vi "measure_mpps.vi"(0 "User Name":string, 1 "Cell details cluster":T2={"Cell Position"=16, "Cell Label"="", "Pixel to measure"=0, "Area (cm^2)"=0.126, "Variable"="", "Variable value"="", "Scan settings in queue"=0, "Light or dark"="", "Measurement Type"=""} {"Pixel to measure" items=["All", "1", "2", "3", "4", "5", "6", "7", "8"]}, 3 "Date array":string[](array[string]), 5 "Experiment Title":string, 9 "File path of JV log":path, 11 "Intensity (no. of suns)":string, 12 "Scan settings":T1={"J-V scan"=TRUE, "Start voltage (V)"=0.0, "End voltage (V)"=0.0, "Step voltage (V)"=1.4, "Scan both directions"=TRUE, "Inverted device structure"=FALSE, "Measurement delay (s)"=10.0, "Measurement speed"=0, "Scan rate (V/s)"=0.0, "Stabilisation time (s)"=0.0, "Stabilisation mode"=0, "Stabilisation value (V or A) "=1.0, "Illumination"=0, "Stabilisation in the dark?"=FALSE, "Repeat light scans"=FALSE, "No. of repeat scans"=0.0, "Only repeat for best pixel"=1, "J-t scan"=FALSE, "J-t best pixel only"=7, "J-t start voltage (V)"=0.0, "J-t end voltage (V)"=1.4, "J-t step voltage (V)"=0.01, "Step time (s)"=0.7, "J-t scan both directions"=TRUE, "J-t inverted device structure"=FALSE, "Settling delay (s)"=0.0, "J-t measurement speed"=0, "J-t illumination"=2, "Max. power stabilisation"=FALSE, "Max power best pixel only"=1, "Max. power point tracker"=FALSE, "Vmp from J-V scan"=FALSE, "Max P stab. Specific voltage"=FALSE, "Vmp (V)"=1.0, "Stabilisation time step (s)"=1.0, "Total stabilisation time (s)"=100.0} {"Settling delay (s)" min=0.0; "J-t illumination" items=["Light only", "Dark only", "Light then dark", "Dark then light"]; "Measurement speed" items=["Fast", "Normal", "High accuracy"]; "Illumination" items=["Light only", "Dark only", "Light then dark", "Dark then light"]; "Only repeat for best pixel" items=["only for best pixel", "for best 2 pixels", "for best 3 pixels", "for best 4 pixels", "for best 5 pixels", "for best 6 pixels", "for best 7 pixels", "for all pixels"]; "No. of repeat scans" min=1.0 step=1.0; "Max power best pixel only" items=["only the best pixel", "the best 2 pixels", "the best 3 pixels", "the best 4 pixels", "the best 5 pixels", "the best 6 pixels", "the best 7 pixels", "all pixels"]; "J-t best pixel only" items=["only the best pixel", "the best 2 pixels", "the best 3 pixels", "the best 4 pixels", "the best 5 pixels", "the best 6 pixels", "the best 7 pixels", "all pixels"]; "J-t measurement speed" items=["Fast", "Normal", "High Accuracy"]; "Stabilisation mode" items=["V", "I"]; "Measurement delay (s)" min=0.01}, 13 "VISA resource name":refnum<visa-resource-name>="GPIB1::24::INSTR", 14 "Skip pixel?":bool) -> (4 "Jt Curve":cluster{"Y":dbl[], "Y":dbl[]}[](graph) caption="JV Curve")   [LabVIEW 2016]
uses:
  TypeDefs/scan_settings.ctl
  <vilib>/Utility/file.llb/Read Delimited Spreadsheet (DBL).vi
panel:
  out "VISA resource name 2":refnum<visa-resource-name>="GPIB1::24::INSTR"
  out "File path for Jt image":path
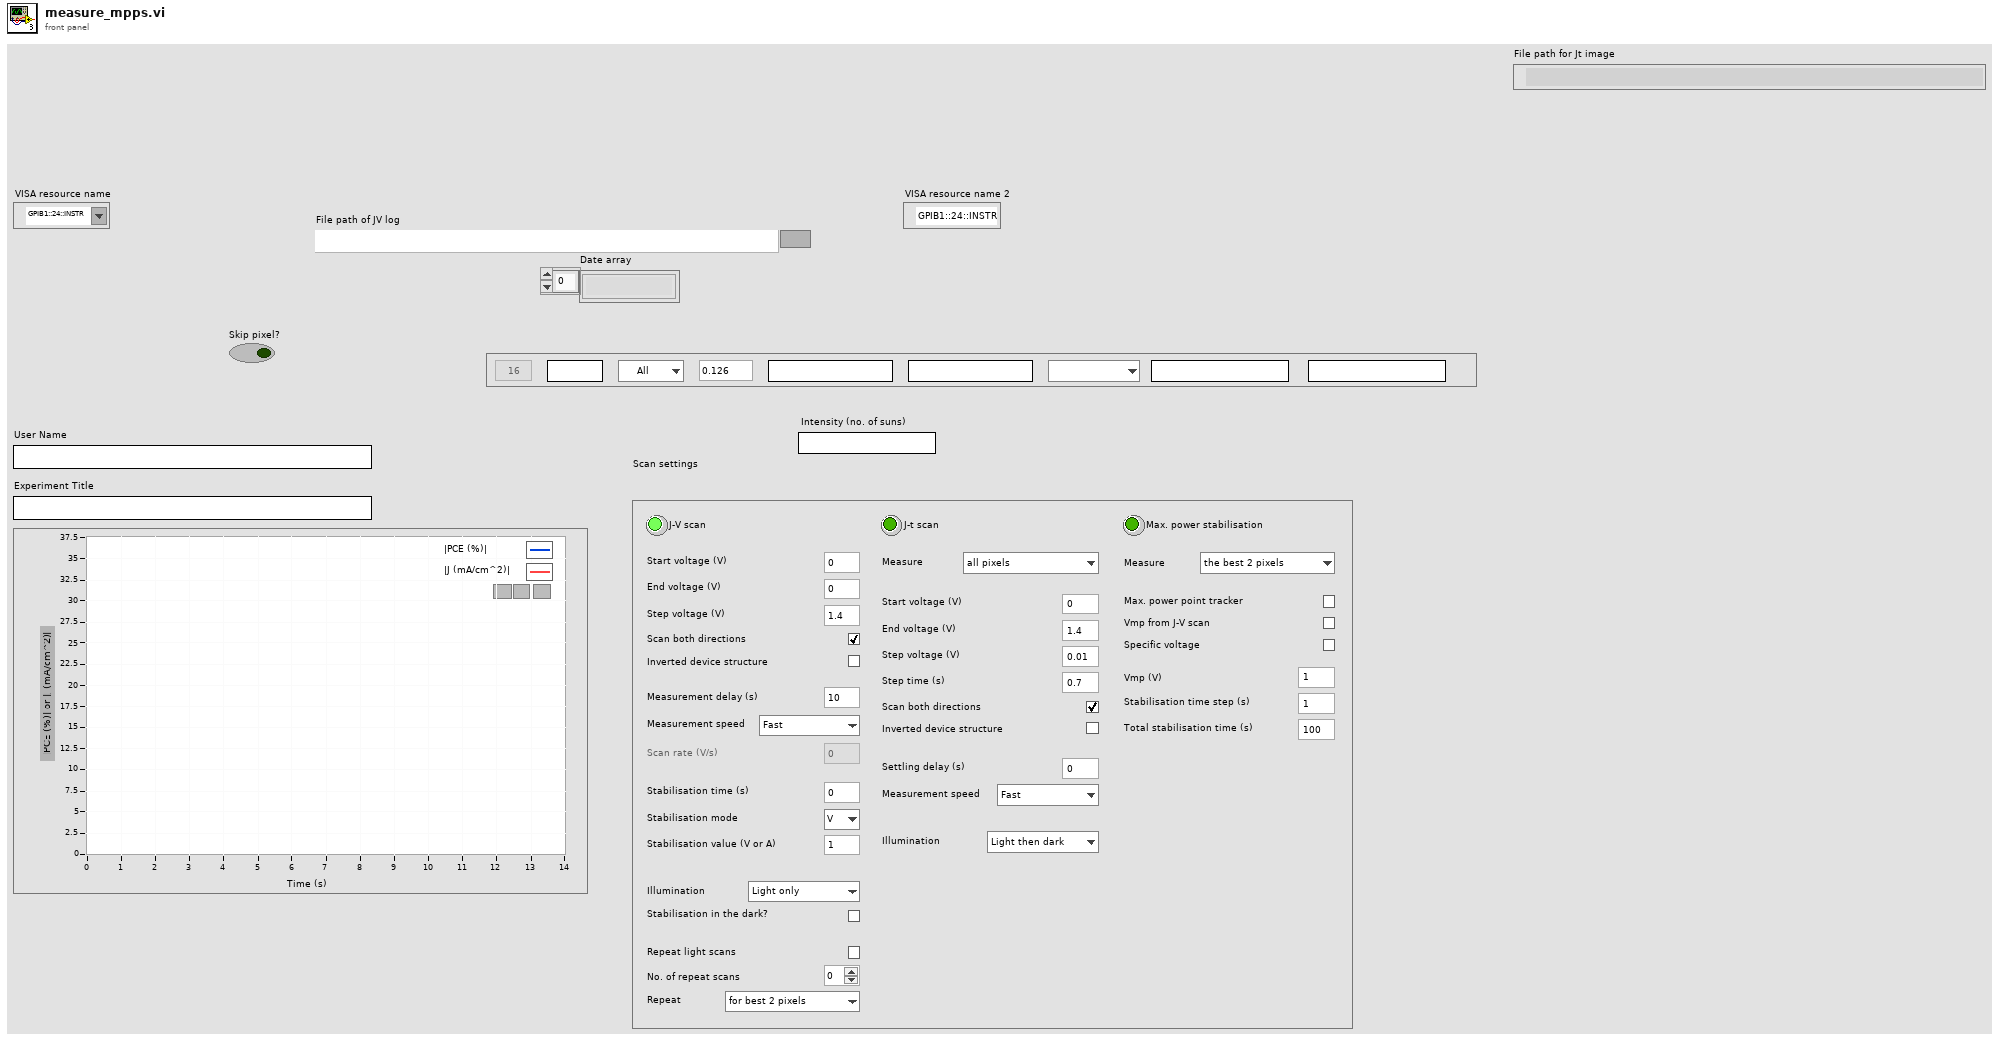
[diagram p1: front panel]
types:
  T1 = typedef "scan_settings.ctl" = cluster{"J-V scan":bool, "Start voltage (V)":dbl, "End voltage (V)":dbl, "Step voltage (V)":dbl, "Scan both directions":bool, "Inverted device structure":bool, "Measurement delay (s)":dbl, "Measurement speed":u8, "Scan rate (V/s)":dbl, "Stabilisation time (s)":dbl, "Stabilisation mode":u16, "Stabilisation value (V or A) ":dbl, "Illumination":u16, "Stabilisation in the dark?":bool, "Repeat light scans":bool, "No. of repeat scans":dbl, "Only repeat for best pixel":u16, "J-t scan":bool, "J-t best pixel only":u16, "J-t start voltage (V)":dbl, "J-t end voltage (V)":dbl, "J-t step voltage (V)":dbl, "Step time (s)":dbl, "J-t scan both directions":bool, "J-t inverted device structure":bool, "Settling delay (s)":dbl, "J-t measurement speed":u16, "J-t illumination":u16, "Max. power stabilisation":bool, "Max power best pixel only":u16, "Max. power point tracker":bool, "Vmp from J-V scan":bool, "Max P stab. Specific voltage":bool, "Vmp (V)":dbl, "Stabilisation time step (s)":dbl, "Total stabilisation time (s)":dbl}
  T2 = cluster{"Cell Position":i32, "Cell Label":string, "Pixel to measure":u16, "Area (cm^2)":dbl, "Variable":string, "Variable value":string, "Scan settings in queue":u16, "Light or dark":string, "Measurement Type":string}
  T3 = typedef "imagedata.ctl" = cluster{"image type":i32, "image depth":i32, "image":u8[], "mask":u8[], "colors":u32[], "Rectangle":cluster{"left":i16, "top":i16, "right":i16, "bottom":i16}}
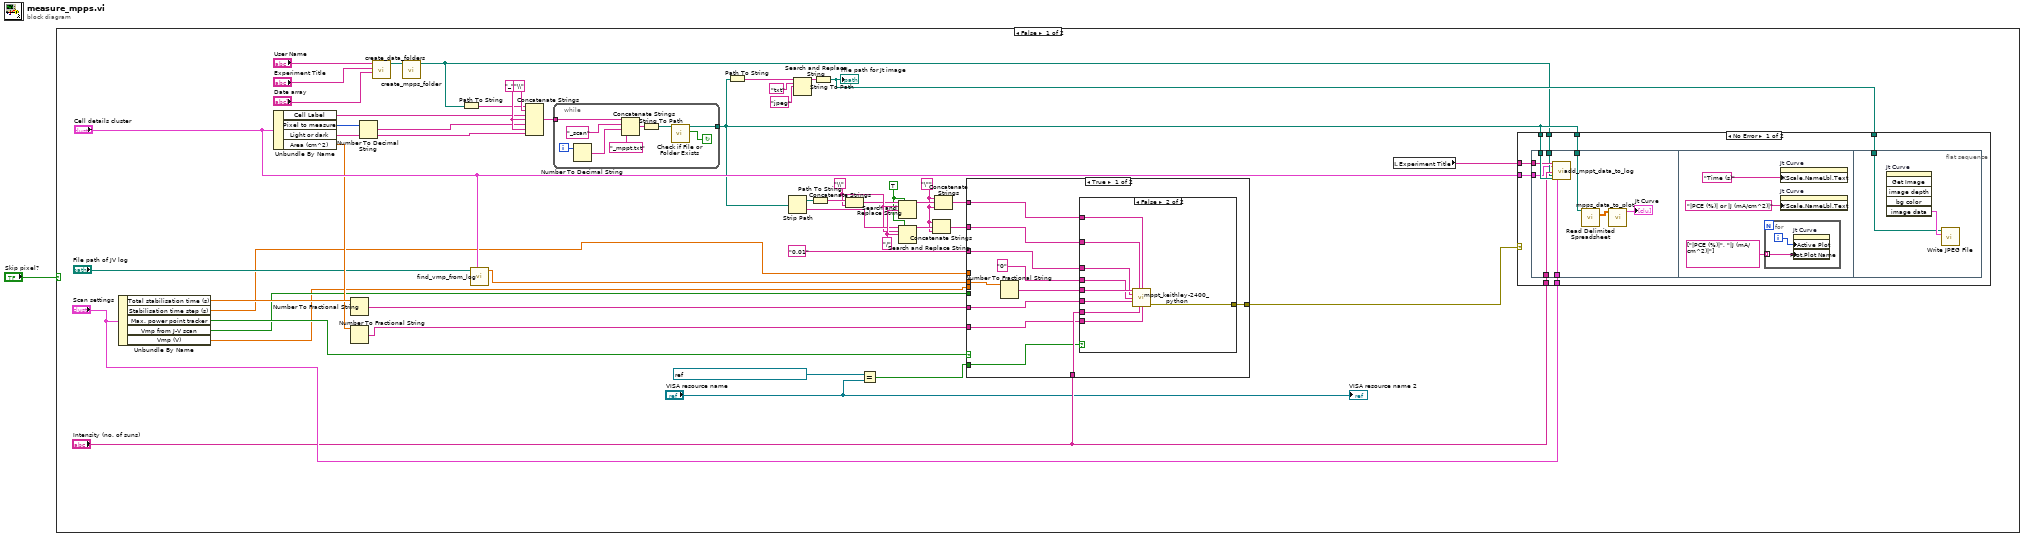
[diagram p0: block diagram]
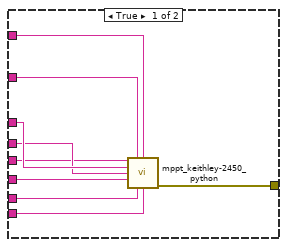
[diagram p2: hidden frame]
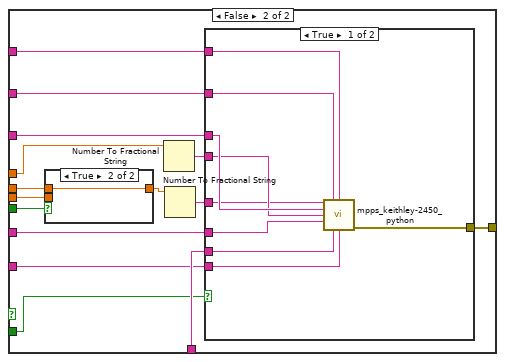
[diagram p3: hidden frame]
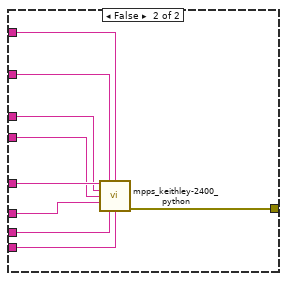
[diagram p5: hidden frame]
diagram:
  n1 = case shown="False" "Skip pixel?" {
    frame False {
      w22 = "\"" ("string")
      w13 = TRUE ("replace all? (F)")
      w33 = "/" ("search string")
      w21 = "\\" ("search string")
      w42 = "_"
      n2 = Unbundle By Name("Scan settings") -> ("Total stabilisation time (s)"=w49:dbl, "Stabilisation time step (s)"=w5:dbl, "Max. power point tracker"=w9:bool, "Vmp from J-V scan"=w8:bool, "Vmp (V)"=w6:dbl)
      n3 = Unbundle By Name("Cell details cluster") -> ("Cell Label"=w38:string, "Pixel to measure"=w39:u16, "Light or dark"=w36:string, "Area (cm^2)"=w30:dbl)
      n4 = Number To Fractional String(number=w30) -> (F-format string=w19:string)  [unwired: 3 in]
      n5 = Number To Fractional String(number=w49) -> (F-format string=w18:string)  [unwired: 3 in]
      n6 = Number To Decimal String(number=w39) -> (decimal integer string=w37:string)  [unwired: 1 in]
      n7 = call "create_data_folders.vi"("Date array"="Date array", "Experiment Indicator"="Experiment Title", "username"="User Name") -> ("Data Output Folder"=w43:path)  [unwired: 8 in]
      n8 = call "create_mpps_folder.vi"("Data Folder In"=w43) -> ("Data Output Folder"=w23:path)  [unwired: 10 in]
      n9 = Path To String(path=w23) -> (string=w34:string)
      n10 = call "find_vmp_from_log.vi"("Cell details cluster in"="Cell details cluster", "File path of JV log"="File path of JV log") -> ("Vmp"=w7:dbl)  [unwired: 9 in]
      n11 = Concatenate Strings(w34, "\\", w38, w42, w37, w42, w36) -> (w41:string)
      n12 = while {
        tunnel: w41 -> [w148]
        tunnel: [w140] -> w25
        i -> [w146]
        stop <- w141 continue-if-true
        n13 = Number To Decimal String(number=w146) -> (decimal integer string=w145:string)  [unwired: 1 in]
        n14 = Concatenate Strings(w148, "_scan", w145, "_mppt.txt") -> (w142:string)
        n15 = String To Path(string=w142) -> (path=w143:path)
        n16 = call <vilib>:"Check if File or Folder Exists.vi"("path"=w143) -> ("file or folder exists?"=w141:bool, "dup path"=w140:path)  [unwired: 8 in, 1 out]
      }
      n17 = Path To String(path=w25) -> (string=w47:string)
      n18 = Strip Path(path=w25) -> (stripped path=w28:path, name=w29:string)
      n19 = Search and Replace String(input string=w47, search string="txt", replace string="jpeg") -> (result string=w44:string)  [unwired: 5 in, 3 out]
      n20 = Path To String(path=w28) -> (string=w27:string)
      n21 = String To Path(string=w44) -> (path=w31:path)
      "File path for Jt image" <- w31
      n22 = Concatenate Strings(w27, w21) -> (w14:string)
      n23 = Equal?(x=refnum<visa-resource-name> "USB0::0x05E6::0x2450::04049675::INSTR", y="VISA resource name") -> (x = y?=w2:bool)
      n24 = Search and Replace String(replace all?=w13, input string=w29, search string=w21, replace string=w33) -> (result string=w32:string)  [unwired: 4 in, 3 out]
      n25 = Search and Replace String(replace all?=w13, input string=w14, search string=w21, replace string=w33) -> (result string=w35:string)  [unwired: 4 in, 3 out]
      n26 = Concatenate Strings(w22, w32, w22) -> (w16:string)
      n27 = Concatenate Strings(w22, w35, w22) -> (w17:string)
      n28 = case shown="True" w9 {
        tunnel: "Intensity (no. of suns)" -> [w62 w95]
        tunnel: [w61 w94] -> w20
        tunnel: w19 -> [w60 w93]
        tunnel: w18 -> [w59 w92]
        tunnel: w17 -> [w58 w91]
        tunnel: w16 -> [w57 w90]
        tunnel: "0.01" ("search string") -> [w56 w89]
        tunnel: w2 -> [w55 w81]
        tunnel: w8 -> [_ w87]
        tunnel: w7 -> [w54 w85]
        tunnel: w6 -> [_ w84]
        tunnel: w5 -> [_ w82]
        frame True {
          n29 = Number To Fractional String(number=w54) -> (F-format string=w53:string)  [unwired: 3 in]
          n30 = case shown="False" w55 {
            tunnel: [w71 w80] -> w61
            tunnel: w62 -> [w64 w79]
            tunnel: w60 -> [w63 w78]
            tunnel: w59 -> [w65 w77]
            tunnel: w53 -> [w66 w76]
            tunnel: w58 -> [w70 w75]
            tunnel: w57 -> [w69 w74]
            tunnel: w56 -> [w68 w73]
            tunnel: "0" ("search string") -> [w67 w72]
            frame True {
              n31 = call "mppt_keithley-2450_python.vi"("start voltage (V)"=w66, "file name"=w69, "folder path"=w70, "nplc"=w68, "settling delay (s)"=w67, "total tracking time (s)"=w65, "illumination intensity (suns equiv.)"=w64, "area (cm^2)"=w63) -> ("error out"=w71:errorcluster)  [unwired: 7 in]
            }
            frame False {
              n32 = call "mppt_keithley-2400_python.vi"("start voltage (V)"=w76, "file name"=w74, "folder path"=w75, "nplc"=w73, "settling delay (s)"=w72, "total tracking time (s)"=w77, "illumination intensity (suns equiv.)"=w79, "area (cm^2)"=w78) -> ("error out"=w80:errorcluster)  [unwired: 7 in]
            }
          }
        }
        frame False {
          n33 = case shown="True" w87 {
            tunnel: [w96 w97] -> w86
            tunnel: w85 -> [_ w97]
            tunnel: w84 -> [w96 _]
            frame False {
            }
            frame True {
            }
          }
          n34 = Number To Fractional String(number=w82) -> (F-format string=w83:string)  [unwired: 3 in]
          n35 = Number To Fractional String(number=w86) -> (F-format string=w88:string)  [unwired: 3 in]
          n36 = case shown="True" w81 {
            tunnel: [w106 w115] -> w94
            tunnel: w95 -> [w99 w114]
            tunnel: w93 -> [w98 w113]
            tunnel: w92 -> [w100 w112]
            tunnel: w88 -> [w101 w111]
            tunnel: w91 -> [w105 w110]
            tunnel: w90 -> [w104 w109]
            tunnel: w89 -> [w103 w108]
            tunnel: w83 -> [w102 w107]
            frame True {
              n37 = call "mpps_keithley-2450_python.vi"("start voltage (V)"=w101, "file name"=w104, "folder path"=w105, "nplc"=w103, "settling delay (s)"=w102, "total tracking time (s)"=w100, "illumination intensity (suns equiv.)"=w99, "area (cm^2)"=w98) -> ("error out"=w106:errorcluster)  [unwired: 7 in]
            }
            frame False {
              n38 = call "mpps_keithley-2400_python.vi"("start voltage (V)"=w111, "file name"=w109, "folder path"=w110, "nplc"=w108, "settling delay (s)"=w107, "total tracking time (s)"=w112, "illumination intensity (suns equiv.)"=w114, "area (cm^2)"=w113) -> ("error out"=w115:errorcluster)  [unwired: 7 in]
            }
          }
        }
      }
      n39 = local read "Experiment Title"() -> (w24:string)
      n40 = case shown="No Error" w20 {
        tunnel: w25 -> [w123 _]
        tunnel: w31 -> [w122 _]
        tunnel: "Scan settings" -> [w121 _]
        tunnel: w25 -> [w120 _]
        tunnel: "Intensity (no. of suns)" -> [w119 _]
        tunnel: w24 -> [w118 _]
        tunnel: w23 -> [w117 _]
        tunnel: "Cell details cluster" -> [w116 _]
        frame No Error {
          n41 = flat-sequence {
            tunnel: w123 -> [w132]
            tunnel: w121 -> [w130]
            tunnel: w120 -> [w129]
            tunnel: w119 -> [w128]
            tunnel: w118 -> [w127]
            tunnel: w117 -> [w126]
            tunnel: w116 -> [w125]
            tunnel: w122 -> [w138]
            frame #0 {
              n42 = call "add_mppt_data_to_log.vi"("Experiment Indicator"=w127, "Cell details cluster"=w125, "Intensity (no. of suns)"=w128, "mppt folder path"=w126, "mppt file path"=w129, "Scan settings"=w130) -> ()  [unwired: 12 in, 2 out]
              n43 = call-poly <vilib>:"Read Delimited Spreadsheet.vi"("file path (dialog if empty)"=w132) -> ("all rows"=w131:dbl[][])  [unwired: 9 in, 5 out]
              n44 = call "mpps_data_to_plot.vi"("Data Array"=w131) -> ("JV Curve"=→"Jt Curve":cluster{"Y":dbl[], "Y":dbl[]}[])  [unwired: 10 in]
            }
            frame #1 {
              n45 = for {
                tunnel: string[] ["|PCE (%)|", "|J (mA/cm^2)|"] ("Measurement queue") -> [w136] mode=indexing
                i -> [w137]
                n46 = property on="Jt Curve" class="XYGraph (strict)"("Active Plot"=w137, "Plot.Plot Name"=w136) -> ()  [unwired: 2 in, 2 out]
              }
              n47 = property on="Jt Curve" class="XYGraph (strict)"("XScale.NameLbl.Text"="Time (s)" ("Y Scale.Name Label.Text")) -> ()  [unwired: 2 in, 2 out]
              n48 = property on="Jt Curve" class="XYGraph (strict)"("YScale.NameLbl.Text"="|PCE (%)| or |J (mA/cm^2)|" ("Y Scale.Name Label.Text")) -> ()  [unwired: 2 in, 2 out]
            }
            frame #2 {
              n49 = invoke on="Jt Curve" class="XYGraph (strict)" method="Get Image"() -> ("image data"=w139:T3)  [unwired: 6 in, 5 out]
              n50 = call <vilib>:"Write JPEG File.vi"("image data"=w139, "path to JPEG file"=w138) -> ()  [unwired: 8 in, 2 out]
            }
          }
        }
        frame Error {
        }
      }
      "VISA resource name 2" <- "VISA resource name"
    }
    frame True {
    }
  }
